vi "RPC_Create.vi"(0 "reference in":refnum<class "RPC.lvclass">, 5 "error in (no error)":errorcluster, 6 "Time Data IN":refnum<class "GSwFormDSP.lvclass">, 7 "Application Name":string, 9 "State Queue":string[](array[string])) -> (14 "reference out":refnum<class "RPC.lvclass">, 19 "error out":errorcluster)   [LabVIEW 2022 SP3, in "RPC.lvclass"]
doc: "Constructor."
uses:
  RPC.lvclass
  C:/Program Files/National Instruments/LabVIEW 2022/vi.lib/addons/_AddQ/G#Object/G#Object.lvclass
  W:/projects/archives/23 Charette AI Group/SPWB/API/Generic Utilities_class/Generic Utilities.lvclass
  API/GSwFormDSP_class/GSwFormDSP.lvclass
  <vilib>/addons/_AddQ/G#Object/G#Object.lvclass
  API/Generic Utilities_class/Generic Utilities.lvclass
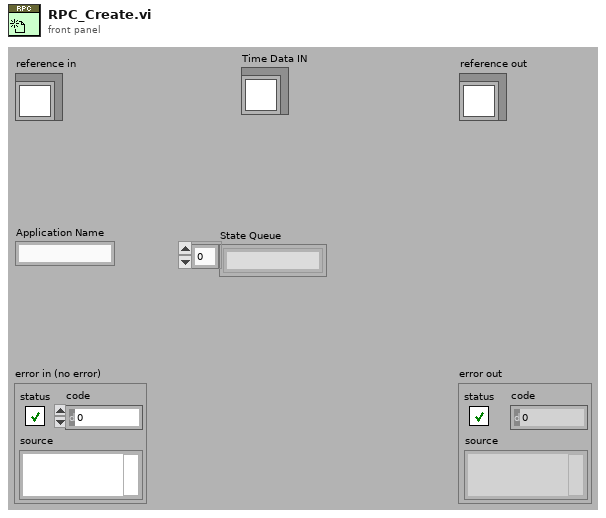
[diagram p1: front panel]
types:
  T1 = typedef "RPC.lvclass/ObjectAttributesRef.ctl" = refnum<data-value>
  T2 = typedef "RPC.lvclass/ObjectAttributes.ctl" = cluster{"File Refnum":refnum<file>, "File total size":i32, "Offset from start of file":i32, "Time Type":enum16{"Response", "Drive"}, "Full Scale":dbl[unit], "New Time Data Obj?":bool, "Header":cluster{"Num Header":i32, "Num Parameter":i32, "Nb Channels":i32, "dT":dbl, "Number of Groups":i32, "Group size":i32, "Units":string[], "Names":string[], "Sensitivity":dbl[], "Complete header":string[]}, "Time Data":refnum<class "GSwFormDSP.lvclass">}
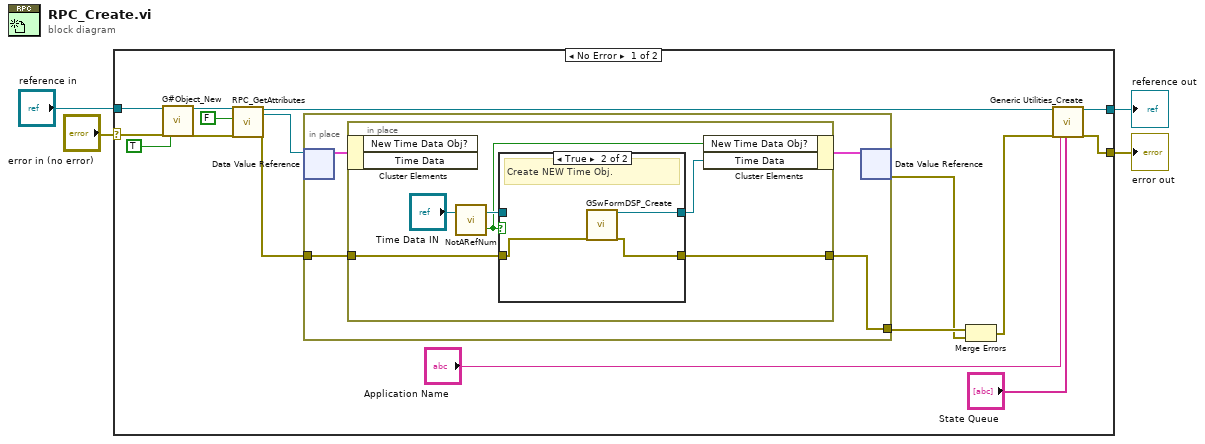
[diagram p0: block diagram]
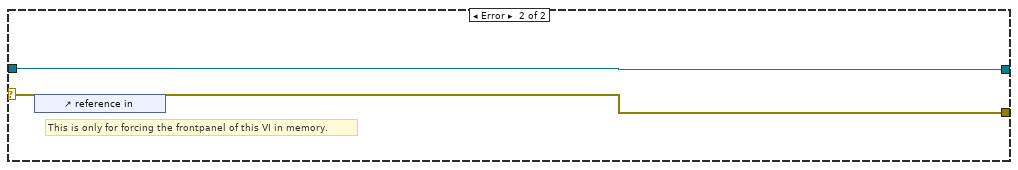
[diagram p3: hidden frame]
diagram:
  n1 = case shown="No Error" "error in (no error)" {
    selector: "error in (no error)" -> [w19 w37]
    tunnel: [w8 w37] -> w3
    tunnel: [w10 w36] -> w1
    tunnel: "reference in" -> [w20 w36]
    frame No Error {
      n2 = call <vilib>:"G#Object_New.vi"("reference in"=w20, "error in (no error)"=w19, "user counter (T)?"=TRUE ("User Counter")) -> ("reference out"=w13:refnum<class "RPC.lvclass">, "error out"=w12:errorcluster)  [unwired: 14 in, 1 out]
      n3 = call "RPC_GetAttributes.vi"("reference in"=w13, "return data? (T)"=FALSE ("return data"), "error in (no error)"=w12) -> ("reference out"=w11:refnum<class "RPC.lvclass">, "attributes ref"=w15:T1, "error out"=w6:errorcluster)  [unwired: 13 in, 1 out]
      n4 = in-place {
        in-place-border: [w21] -> w17
        in-place-border: w6 -> [w22]
        n5 = in-place-dvr #1(w15) -> (w23:T2)  [unwired: 1 out]
        n6 = in-place {
          in-place-border: w22 -> [w28]
          in-place-border: [w27] -> w21
          n7 = in-place-cluster #2(w23) -> ()  [unwired: 2 out]
          n8 = call-dynamic "NotARefNum.vi"("reference in"="Time Data IN") -> ("not a refnum?"=w25:bool, "reference out"=w30:refnum<class "GSwFormDSP.lvclass">)  [unwired: 1 in]
          n9 = case shown="True" w25 {
            tunnel: [w32 w35] -> w26
            tunnel: w30 -> [w32 _]
            tunnel: w28 -> [w31 w34]
            tunnel: [w31 w33] -> w27
            frame False {
              # "Copy an existing reference."
            }
            frame True {
              # "Create NEW Time Obj."
              n10 = call "GSwFormDSP_Create.vi"("error in (no error)"=w34) -> ("reference out"=w35:refnum<class "GSwFormDSP.lvclass">, "error out"=w33:errorcluster)  [unwired: 17 in]
            }
          }
          n11 = in-place-cluster #2("New Time Data Obj?"=w25, "Time Data"=w26) -> (w24:T2)
        }
        n12 = in-place-dvr #1(w24) -> (w16:errorcluster)  [unwired: 1 out]
      }
      n13 = Merge Errors(w17, w16) -> (w9:errorcluster)
      n14 = call "Generic Utilities_Create.vi"("reference in"=w11, "error in (no error)"=w9, "Application Name"="Application Name", "State Queue"="State Queue") -> ("reference out"=w10:refnum<class "RPC.lvclass">, "error out"=w8:errorcluster)  [unwired: 14 in]
    }
    frame Error {
      # "This is only for forcing the frontpanel of this VI in memory."
      n15 = control-ref of="reference in"() -> ()  [unwired: 1 out]
    }
  }
  "error out" <- w3
  "reference out" <- w1
